vi "Validate Incoming Packet.vi"(8 "error in (no error)":errorcluster, 10 "ControlPacket":refnum<class "ControlPacket.lvclass">, 11 "Session in":refnum<class "Session.lvclass">) -> (0 "error out":errorcluster, 1 "Protocol Violation":bool, 2 "ControlPacket out":refnum<class "ControlPacket.lvclass">, 3 "Session out":refnum<class "Session.lvclass">)   [LabVIEW 2013, in "MQTT Server.lvlib" / "Session.lvclass"]
uses:
  Session.lvclass
  Control Packets/ControlPacket/ControlPacket.lvclass
  Session.lvclass/Session.ctl
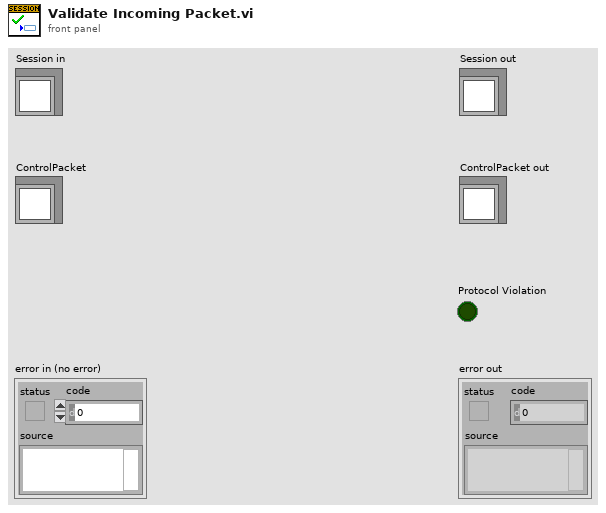
[diagram p1: front panel]
types:
  T1 = typedef "ControlPacket.lvclass/Control Packet Type -- enum.ctl" = enum16{"Reserved", "CONNECT", "CONNACK", "PUBLISH", "PUBACK", "PUBREC", "PUBREL", "PUBCOMP", "SUBSCRIBE", "SUBACK", "UNSUBSCRIBE", "UNSUBACK", "PINGREQ", "PINGRESP", "DISCONNECT", "Reserved(15)"}
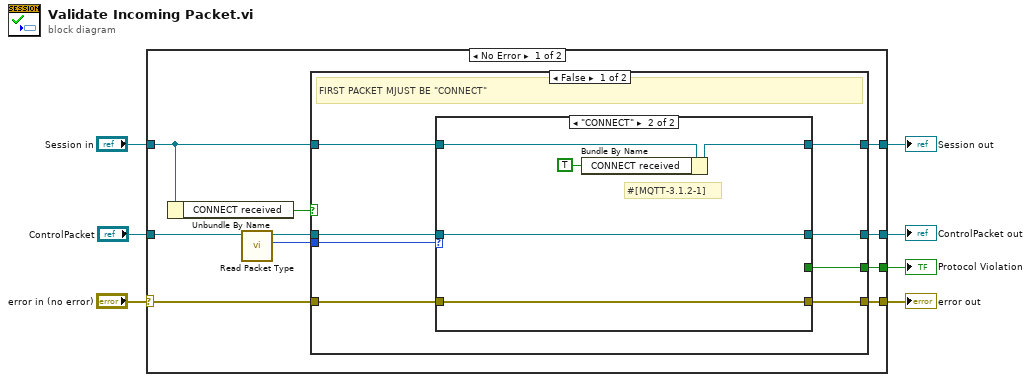
[diagram p0: block diagram]
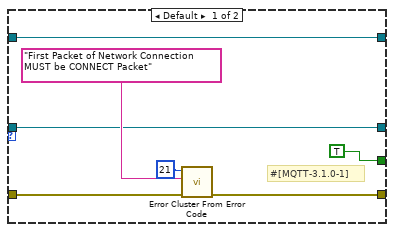
[diagram p2: hidden frame]
diagram:
  n1 = case shown="No Error" "error in (no error)" {
    selector: "error in (no error)" -> [w10 w43]
    tunnel: [w9 w43] -> w6
    tunnel: [w11 w42] -> w4
    tunnel: "Session in" -> [w15 w42]
    tunnel: "ControlPacket" -> [w14 w41]
    tunnel: [w17 w41] -> w2
    tunnel: [w8 _] -> w1
    frame No Error {
      n2 = Unbundle By Name(w15) -> ("CONNECT received"=w16:bool)
      n3 = call "Read Packet Type.vi"("ControlPacket in"=w14) -> ("Control Packet Type"=w12:T1, "ControlPacket out"=w13:refnum<class "ControlPacket.lvclass">)  [unwired: 9 in]
      n4 = case shown="False" w16 {
        tunnel: w13 -> [w19 w40]
        tunnel: [w20 w40] -> w17
        tunnel: w15 -> [w22 w39]
        tunnel: w12 -> [w23 _]
        tunnel: [w21 w39] -> w11
        tunnel: w10 -> [w25 w38]
        tunnel: [w24 w38] -> w9
        tunnel: [w18 _] -> w8
        frame False {
          # "FIRST PACKET MJUST BE \"CONNECT\""
          n5 = case shown="\"CONNECT\"" w23 {
            tunnel: w25 -> [w31 w33]
            tunnel: [w32 w33] -> w24
            tunnel: w22 -> [w27 w37]
            tunnel: [w27 w36] -> w21
            tunnel: [w28 w34] -> w20
            tunnel: w19 -> [w28 w34]
            tunnel: [TRUE _] -> w18
            frame Default {
              # "#[MQTT-3.1.0-1]"
              n6 = call <vilib>:"Error Cluster From Error Code.vi"("error in (no error)"=w31, "error message (\"\")"="First Packet of Network Connection MUST be CONNECT Packet", "error code (0)"=21) -> ("error out"=w32:errorcluster)  [unwired: 6 in]
            }
            frame "CONNECT" {
              # "#[MQTT-3.1.2-1]"
              n7 = Bundle By Name(cluster=w37, "CONNECT received"=TRUE) -> (w36:refnum<class "Session.lvclass">)
            }
          }
        }
        frame True {
        }
      }
    }
    frame Error {
    }
  }
  "error out" <- w6
  "Session out" <- w4
  "ControlPacket out" <- w2
  "Protocol Violation" <- w1
